vi "WPI_CameraRead MJPG for Dashboard.vi"(6 "Camera Settings":T6={"fps"=30, "compression"=30, "Image Size"=enum."320x240", "Config Shown"=FALSE}, 7 "Camera Settings 2":T3={"Exposure"=enum."Auto", "Exposure (%)"=50.0, "Brightness"=50, "White Balance"=enum."Auto", "Color Temp (K)"=0.0} {"Brightness" min=0 max=100}, 8 "Rec Mode":u16(ring) items=["Stop", "Record", "Playback Panel"], 9 "NT Connection":bool, 10 "Capture Info":T5={"Camera Name"="Camera", "Display Name"="left", {"Save Path"=path "", "Interval (s)"=1.0, "Keep"=180}}, 11 "Refnum in":T4) -> (2 "Active":bool, 3 "Refnum out":T4, 4 "FPS":dbl, 5 "Bandwidth (Mbps)":dbl)   [LabVIEW 2017]
doc: "This VI connects to a camera server of the connected robot. It requests images for a given camera name and settings. USB cameras should generally support all settings. IP cameras support only those in Camera Settings cluster. If the settings, name or other settings change, it will close and reopen as needed. The VI should be called repeatedly and it will return with the latest image from the server."
uses:
  <vilib>/Rock Robotics/WPI/Dashboard/WPI_DashboardLogging Global.vi
  <vilib>/Rock Robotics/WPI/Camera/WPI_CameraWhite Balance Values.ctl
  <vilib>/Rock Robotics/WPI/Camera/WPI_CameraExposure Values.ctl
  <vilib>/vision/Image Controls.llb/IMAQ Image.ctl
  <vilib>/Rock Robotics/WPI/Camera/WPI_CameraImageSize.ctl
  <vilib>/Rock Robotics/WPI/Camera/WPI_CameraSettings Read MJPG.ctl
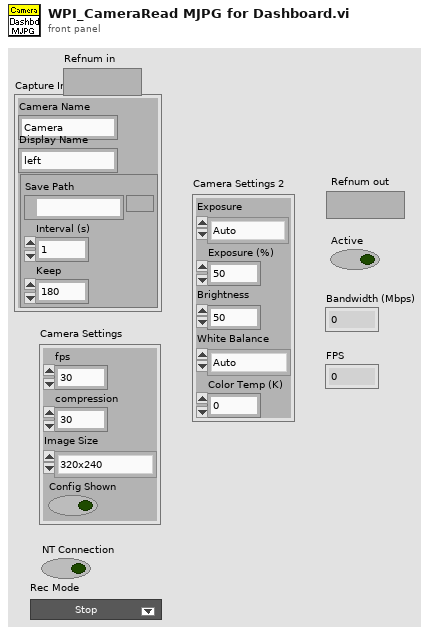
[diagram p1: front panel]
types:
  T1 = typedef "WPI_CameraExposure Values.ctl" = enum16{"Auto", "Flicker-free 50 Hz", "Flicker-free 60 Hz", "Hold current", "Custom"}
  T2 = typedef "WPI_CameraWhite Balance Values.ctl" = enum16{"Auto", "Fixed indoor", "Fixed outdoor 1", "Fixed outdoor 2", "Fixed fluorescent 1", "Fixed fluorescent 2", "Hold current", "Custom"}
  T3 = cluster{"Exposure":T1, "Exposure (%)":dbl, "Brightness":i32, "White Balance":T2, "Color Temp (K)":dbl}
  T4 = typedef "IMAQ Image.ctl" = refnum<image>
  T5 = cluster{"Camera Name":string, "Display Name":string, cluster{"Save Path":path, "Interval (s)":dbl, "Keep":i32}}
  T6 = typedef "WPI_CameraSettings Read MJPG.ctl" = cluster{"fps":i32, "compression":i32, "Image Size":T7, "Config Shown":bool}
  T7 = typedef "WPI_CameraImageSize.ctl" = enum16{"640x480", "320x240", "160x120", "Custom"}
  T8 = cluster{"token string":string, "token string 2":string}[]
  T9 = cluster{"Exposure":bool, "Exposure (%)":bool, "Brightness":bool, "White Balance":bool, "Color Temp (K)":bool}
  T10 = cluster{"token string":string, "token string":string}
  T11 = cluster{"token string":string, "token string":string}[]
  T12 = cluster{"Save Path":path, "Interval (s)":dbl, "Keep":i32}
  T13 = cluster{"Camera Name":string, "fps":i32, "compression":i32, "Image Size":T7}
  T14 = typedef "IMAQ AVI2 Refnum.ctl" = refnum<k20>
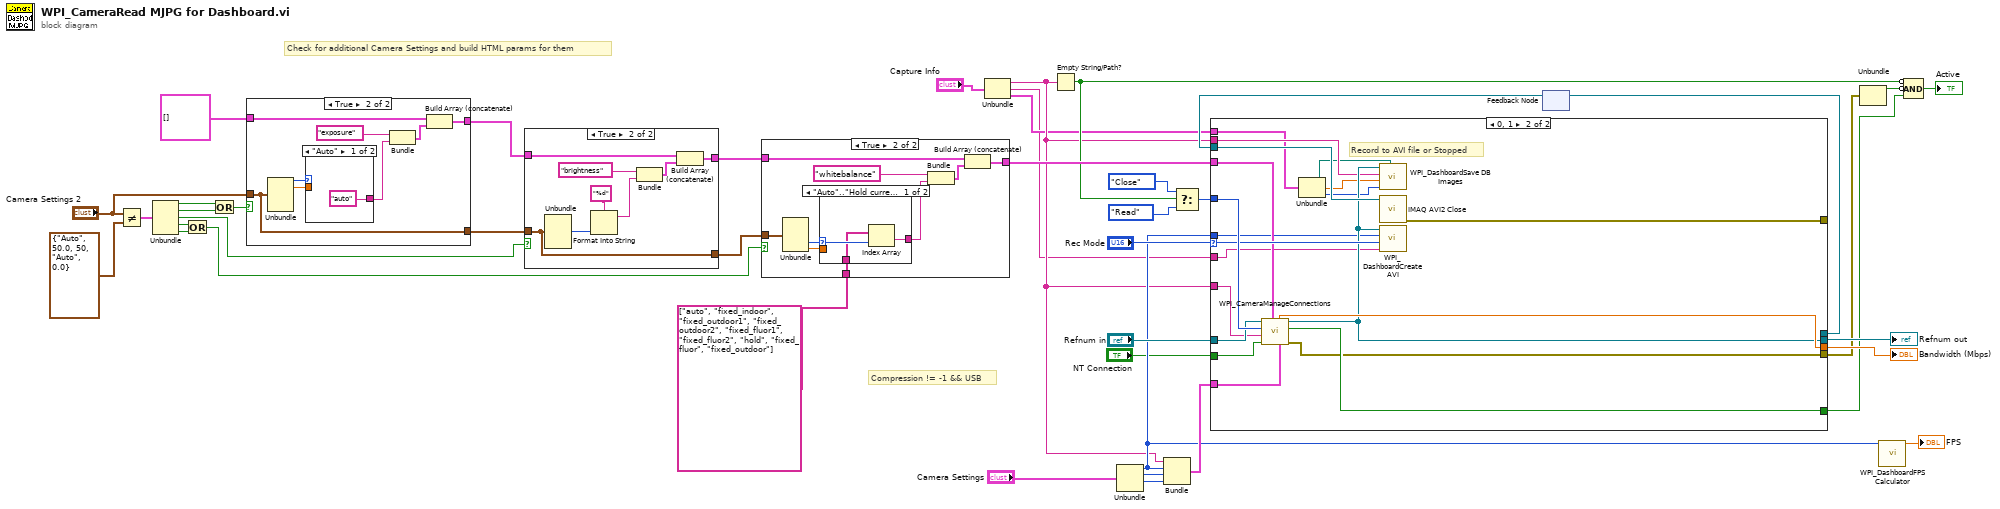
[diagram p0: block diagram]
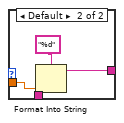
[diagram p3: hidden frame]
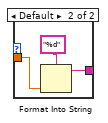
[diagram p6: hidden frame]
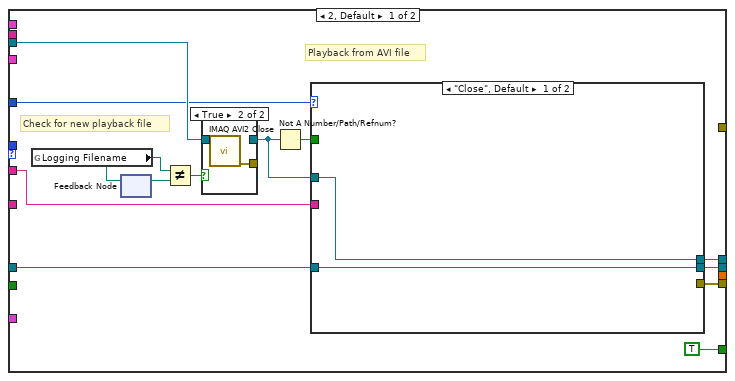
[diagram p7: hidden frame]
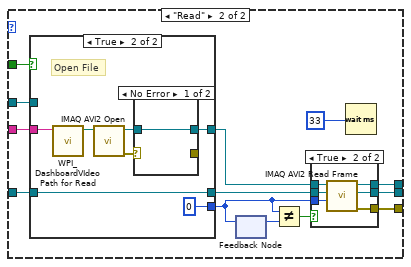
[diagram p9: hidden frame]
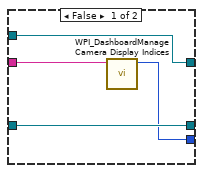
[diagram p11: hidden frame]
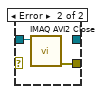
[diagram p12: hidden frame]
diagram:
  # "Check for additional Camera Settings and build HTML params for them"
  # "Compression != -1 && USB"
  n1 = Not Equal?(x="Camera Settings 2", y=T3 {"Exposure"=enum."Auto", "Exposure (%)"=50.0, "Brightness"=50, "White Balance"=enum."Auto", "Color Temp (K)"=0.0} ("Camera Settings 2")) -> (x != y?=w27:T9)
  n2 = Unbundle(w27) -> ("Exposure"=w25:bool, "Exposure (%)"=w24:bool, "Brightness"=w14:bool, "White Balance"=w17:bool, "Color Temp (K)"=w16:bool)
  n3 = Or(x=w17, y=w16) -> (x .or. y?=w15:bool)
  n4 = Or(x=w25, y=w24) -> (x .or. y?=w26:bool)
  n5 = case shown="True" w26 {
    tunnel: "Camera Settings 2" -> [w43 w45]
    tunnel: T8 [] ("parameters") -> [w44 w48]
    tunnel: [w44 w47] -> w22
    tunnel: [w43 w45] -> w19
    frame False {
    }
    frame True {
      n6 = Unbundle(w45) -> ("Exposure"=w51:T1, "Exposure (%)"=w50:dbl)  [unwired: 3 out]
      n7 = case shown="\"Auto\"" w51 {
        tunnel: w50 -> [_ w56]
        tunnel: ["auto" ("token string") w55] -> w49
        frame "Auto" {
        }
        frame Default {
          n8 = Format Into String(format string="%d" ("token string"), w56) -> (resulting string=w55:string)  [unwired: 2 in, 1 out]
        }
      }
      n9 = Bundle("token string"="exposure", "token string"=w49) -> (w46:T10)  [unwired: 1 in]
      n10 = Build Array (concatenate)(w48, w46) -> (w47:T11)
    }
  }
  n11 = case shown="True" w14 {
    tunnel: w19 -> [w57 w60]
    tunnel: w22 -> [w58 w64]
    tunnel: [w58 w63] -> w20
    tunnel: [w57 w60] -> w18
    frame False {
    }
    frame True {
      n12 = Unbundle(w60) -> ("Brightness"=w59:i32)  [unwired: 4 out]
      n13 = Format Into String(format string="%d" ("token string"), w59) -> (resulting string=w65:string)  [unwired: 2 in, 1 out]
      n14 = Bundle("token string"="brightness", w65) -> (w62:cluster{"token string":string, string})  [unwired: 1 in]
      n15 = Build Array (concatenate)(w64, w62) -> (w63:T11)
    }
  }
  n16 = case shown="True" w15 {
    tunnel: w18 -> [_ w75]
    tunnel: w20 -> [w67 w73]
    tunnel: [w67 w72] -> w12
    tunnel: string[] ["auto", "fixed_indoor", "fixed_outdoor1", "fixed_outdoor2", "fixed_fluor1", "fixed_fluor2", "hold", "fixed_fluor", "fixed_outdoor"] ("Array") -> [_ w68]
    frame False {
    }
    frame True {
      n17 = Unbundle(w75) -> ("White Balance"=w70:T2, "Color Temp (K)"=w69:dbl)  [unwired: 3 out]
      n18 = case shown="\"Auto\"..\"Hold current\"" w70 {
        selector: w70 -> [w79 _]
        tunnel: w69 -> [_ w82]
        tunnel: [w78 w81] -> w74
        tunnel: w68 -> [w77 _]
        frame "Auto".."Hold current" {
          n19 = Index Array(array=w77, index=w79) -> (element=w78:string)
        }
        frame Default {
          n20 = Format Into String(format string="%d" ("token string"), w82) -> (resulting string=w81:string)  [unwired: 2 in, 1 out]
        }
      }
      n21 = Bundle("token string"="whitebalance", w74) -> (w71:cluster{"token string":string, string})  [unwired: 1 in]
      n22 = Build Array (concatenate)(w73, w71) -> (w72:T11)
    }
  }
  n23 = Unbundle("Capture Info") -> ("Camera Name"=w3:string, "Display Name"=w1:string, w2:T12)
  n24 = Empty String/Path?(string/path=w3) -> (empty?=w11:bool)
  n25 = Unbundle("Camera Settings") -> ("fps"=w7:i32, "compression"=w10:i32, "Image Size"=w9:T7)  [unwired: 1 out]
  n26 = Bundle("Camera Name"=w3, "fps"=w7, "compression"=w10, "Image Size"=w9) -> (w8:T13)  [unwired: 1 in]
  n27 = Select(t=enum16{"Read", "Reopen", "Close"}."Close" ("Operation"), s=w11, f=enum16{"Read", "Reopen", "Close"}."Read" ("Operation")) -> (s? t:f=w39:enum16{"Read", "Reopen", "Close"})
  n28 = feedback #1() -> (w32:T14)  [unwired: 1 in]
  n29 = case shown="0, 1" "Rec Mode" {
    selector: "Rec Mode" -> [_ w152]
    tunnel: w39 -> [w85 w155]
    tunnel: [_ w154] -> w36
    tunnel: [w95 w149] -> w33
    tunnel: "Refnum in" -> [w93 w153]
    tunnel: w32 -> [w89 w151]
    tunnel: [w92 _] -> w31
    tunnel: [w91 w146] -> w30
    tunnel: [_ w150] -> _
    tunnel: w3 -> [_ w145]
    tunnel: [TRUE w148] -> w28
    tunnel: w12 -> [_ w147]
    tunnel: w8 -> [_ w143]
    tunnel: w7 -> [_ w144]
    tunnel: "NT Connection" -> [_ w142]
    tunnel: w3 -> [_ w141]
    tunnel: w2 -> [_ w140]
    tunnel: w1 -> [w83 w136]
    frame 2, Default {
      # "Check for new playback file"
      # "Playback from AVI file"
      n30 = global read "WPI_DashboardLogging Global.vi" "Logging Filename"() -> (w88:path)
      n31 = feedback #2() -> (w87:path)  [unwired: 1 in]
      n32 = feedback-in #2(w88) -> ()
      n33 = Not Equal?(x=w88, y=w87) -> (x != y?=w86:bool)
      n34 = case shown="True" w86 {
        tunnel: [w96 _] -> w90
        tunnel: w89 -> [w96 w98]
        tunnel: [_ w97] -> _
        frame False {
        }
        frame True {
          n35 = call "IMAQ AVI2 Close"("AVI Refnum"=w98) -> ("error out"=w97:errorcluster)  [unwired: 10 in]
        }
      }
      n36 = Not A Number/Path/Refnum?(number/path/refnum=w90) -> (NaN/Path/Refnum?=w94:bool)
      n37 = case shown="\"Close\", Default" w85 {
        tunnel: [w99 w113] -> w95
        tunnel: w94 -> [_ w112]
        tunnel: w93 -> [w99 w109]
        tunnel: [w100 w108] -> w92
        tunnel: [_ w107] -> w91
        tunnel: w83 -> [_ w106]
        tunnel: w90 -> [w100 w105]
        frame "Close", Default {
        }
        frame "Read" {
          n38 = case shown="True" w112 {
            tunnel: [w125 w130] -> w111
            tunnel: w105 -> [w125 _]
            tunnel: [w124 w132] -> w110
            tunnel: w109 -> [w124 w132]
            tunnel: [w122 0 ("Video Frame #")] -> w102
            tunnel: w106 -> [w123 w127]
            frame False {
              n39 = call <vilib>:"WPI_DashboardManage Camera Display Indices.vi"("Display Name"=w123) -> ("index of element"=w122:i32)  [unwired: 10 in]
            }
            frame True {
              # "Open File"
              n40 = call <vilib>:"WPI_DashboardVIdeo Path for Read.vi"("Display Name"=w127) -> ("Video Path"=w126:path)  [unwired: 10 in]
              n41 = call "IMAQ AVI2 Open"("AVI File Path"=w126) -> ("error out"=w131:errorcluster, "AVI Refnum"=w129:T14)  [unwired: 9 in]
              n42 = case shown="No Error" w131 {
                tunnel: [w133 _] -> w130
                tunnel: w129 -> [w133 w135]
                tunnel: [_ w134] -> _
                frame No Error {
                }
                frame Error {
                  n43 = call "IMAQ AVI2 Close"("AVI Refnum"=w135) -> ("error out"=w134:errorcluster)  [unwired: 10 in]
                }
              }
            }
          }
          n44 = feedback #3() -> (w103:i32)  [unwired: 1 in]
          n45 = feedback-in #3(w102) -> ()
          n46 = Not Equal?(x=w102, y=w103) -> (x != y?=w104:bool)
          n47 = case shown="True" w104 {
            tunnel: [w114 w121] -> w113
            tunnel: w111 -> [w115 w120]
            tunnel: w110 -> [w114 w119]
            tunnel: [w115 w118] -> w108
            tunnel: [_ w117] -> w107
            tunnel: w102 -> [_ w116]
            frame False {
            }
            frame True {
              n48 = call "IMAQ AVI2 Read Frame"("Frame Number"=w116, "Image"=w119, "AVI Refnum"=w120) -> ("error out"=w117:errorcluster, "Image Out"=w121:T4, "AVI Refnum (duplicate)"=w118:T14)  [unwired: 6 in]
            }
          }
          n49 = Wait (ms)(milliseconds to wait=33) -> ()  [unwired: 1 out]
        }
      }
    }
    frame 0, 1 {
      # "Record to AVI file or Stopped"
      n50 = call <vilib>:"WPI_CameraManageConnections.vi"("Cluster"=w143, "parameters"=w147, "NT Connection"=w142, "Camera Name"=w145, "Operation"=w155, "Refnum in"=w153) -> ("error out"=w146:errorcluster, "Active"=w148:bool, "Refnum out"=w149:T4, "Bandwidth (Mbps)"=w154:dbl)  [unwired: 2 in]
      n51 = Unbundle(w140) -> ("Save Path"=w139:path, "Interval (s)"=w138:dbl, "Keep"=w137:i32)
      n52 = call <vilib>:"WPI_DashboardSave DB Images.vi"("Path"=w139, "Images to Keep"=w137, "Time Interval (s)"=w138, "Camera Name"=w141, "Image"=w149) -> ()  [unwired: 5 in]
      n53 = call "IMAQ AVI2 Close"("AVI Refnum"=w151) -> ("error out"=w150:errorcluster)  [unwired: 10 in]
      n54 = call <vilib>:"WPI_DashboardCreate AVI.vi"("Display Name"=w136, "Recording"=w152, "frames per seconds"=w144, "Image"=w149) -> ()  [unwired: 8 in]
    }
  }
  "Bandwidth (Mbps)" <- w36
  "Refnum out" <- w33
  n55 = feedback-in #1(w31) -> ()
  n56 = Unbundle(w30) -> ("status"=w40:bool)  [unwired: 2 out]
  n57 = call <vilib>:"WPI_DashboardFPS Calculator.vi"("Average Count"=w7) -> ("fps"=→"FPS":dbl)  [unwired: 9 in, 1 out]
  n58 = Compound Arithmetic op=AND(invert w11, invert w40, w28) -> (→"Active":bool)
